vi "Initialize Front Panel.vi"(8 "error in (no error)":errorcluster, 11 "ITest Executive Builder Dialog in":refnum<class "ITest Executive Builder Dialog.lvclass">) -> (0 "error out":errorcluster, 3 "ITest Executive Builder Dialog out":refnum<class "ITest Executive Builder Dialog.lvclass">)   [LabVIEW 2017, in "ITest Executive Builder Dialog.lvclass"]
doc: "<License>\nCopyright © 2017 Composed Systems, LLC | All rights reserved\nwww.composed.io\n\nAuthor: Ethan Stern <ethan.stern@composed.io>\n\nThis software is provided \"AS IS\" WITHOUT WARRANTIES, either express or implied, AND IS FOR EDUCATIONAL PURPOSES ONLY.\n</License>"
uses:
  ITest Executive Builder Dialog.lvclass
  <vilib>/gpm_packages/@cs/popup-viewmanager/Source/Popup ViewManager/Popup ViewManager.lvclass
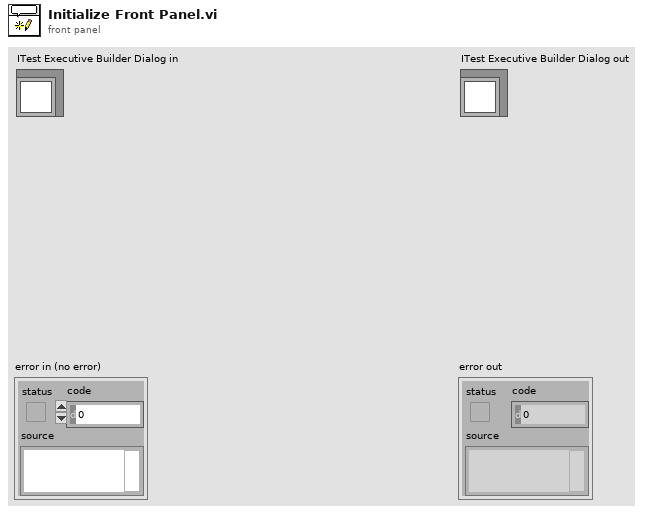
[diagram p1: front panel]
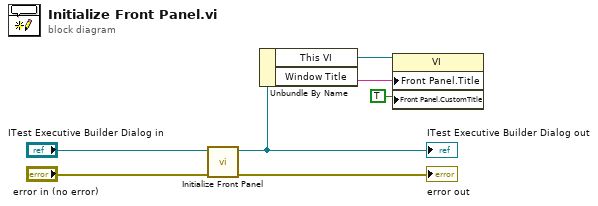
[diagram p0: block diagram]
diagram:
  n1 = call-parent "Initialize Front Panel.vi"("error in (no error)"="error in (no error)", "IViewable in"="ITest Executive Builder Dialog in") -> ("error out"=→"error out":errorcluster, "IViewable out"=w4:refnum<class "ITest Executive Builder Dialog.lvclass">)  [unwired: 8 in]
  "ITest Executive Builder Dialog out" <- w4
  n2 = Unbundle By Name(w4) -> ("This VI"=w3:refnum<vi>, "Window Title"=w2:string)
  n3 = property class="VI"(reference=w3, "Front Panel.Title"=w2, "Front Panel.CustomTitle"=TRUE ("Front Panel Window:Custom Title")) -> ()  [unwired: 1 in, 2 out]
